vi "Feed Snake.vi"(8 "error in (no error)":errorcluster, 10 "Size":u16, 11 "Snake in":refnum<class "Snake.lvclass">) -> (0 "error out":errorcluster, 3 "Snake out":refnum<class "Snake.lvclass">)   [LabVIEW 2021, in "Snake.lvclass"]
uses:
  Snake.lvclass
  C:/Users/poche/Programs/LabVIEW/imposible snake/GameEl_class/GameEl.lvclass
  GameEl_class/GameEl.lvclass/GameEl.ctl
  GameEl_class/GameEl.lvclass
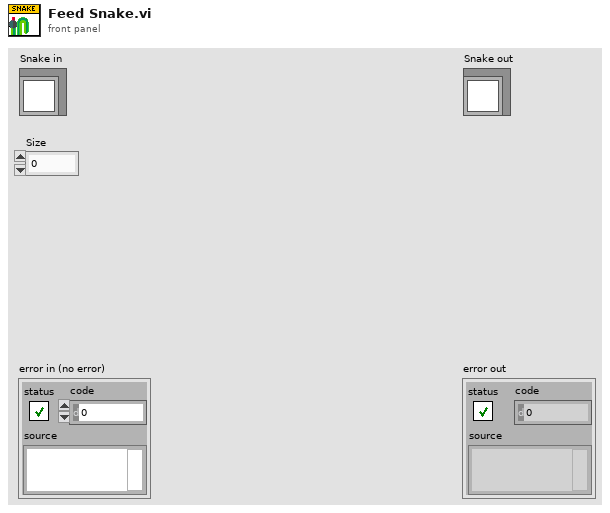
[diagram p1: front panel]
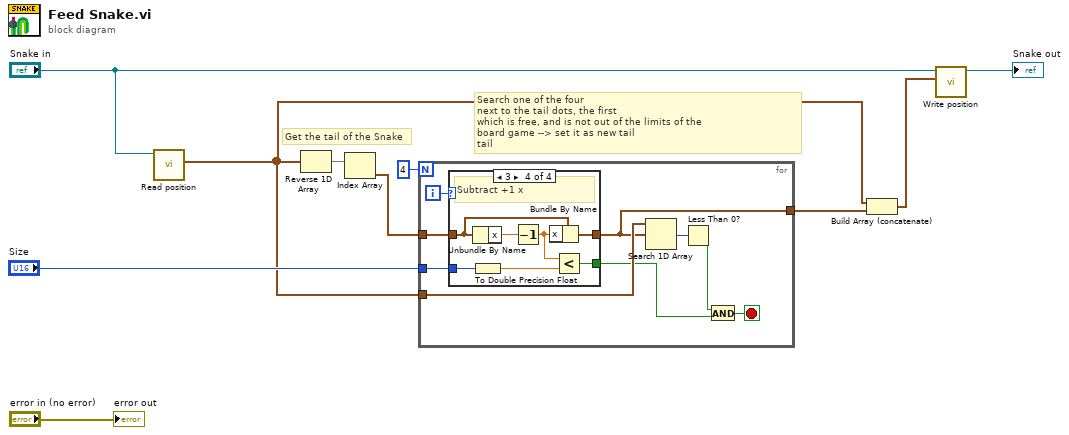
[diagram p0: block diagram]
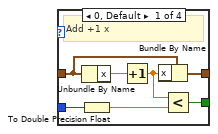
[diagram p2: hidden frame]
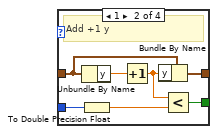
[diagram p3: hidden frame]
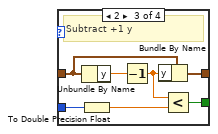
[diagram p4: hidden frame]
diagram:
  # "Search one of the four \nnext to the tail dots, the first \nwhich is free, and is not out of the limits of the \nboard game --> set it as new tail\ntail"
  # "Get the tail of the Snake"
  n1 = call "Read position.vi"("GameEl in"="Snake in") -> ("position"=w4:cluster{"x":dbl, "y":dbl}[])  [unwired: 8 in, 2 out]
  n2 = Reverse 1D Array(array=w4) -> (reversed array=w8:cluster{"x":dbl, "y":dbl}[])
  n3 = Index Array(array=w8) -> (element=w7:cluster{"x":dbl, "y":dbl})  [unwired: 1 in]
  n4 = for {
    N: 4 -> [_]
    tunnel: w7 -> [w19]
    tunnel: w4 -> [w16]
    tunnel: "Size" -> [w17]
    tunnel: [w11] -> w6
    i -> [w18]
    stop <- w12 stop-if-true
    n5 = case shown="3" w18 {
      tunnel: w19 -> [w25 w32 w39 w46]
      tunnel: [w24 w31 w38 w45] -> w11
      tunnel: w17 -> [w22 w29 w36 w43]
      tunnel: [w20 w27 w34 w41] -> w14
      frame 0, Default {
        # "Add +1 x"
        n6 = Unbundle By Name(w25) -> ("x"=w26:dbl)
        n7 = To Double Precision Float(number=w22) -> (double precision float=w21:dbl)
        n8 = Increment(x=w26) -> (x+1=w23:dbl)
        n9 = Bundle By Name(cluster=w25, "x"=w23) -> (w24:cluster{"x":dbl, "y":dbl})
        n10 = Less?(x=w23, y=w21) -> (x < y?=w20:bool)
      }
      frame 1 {
        # "Add +1 y"
        n11 = Unbundle By Name(w32) -> ("y"=w33:dbl)
        n12 = To Double Precision Float(number=w29) -> (double precision float=w28:dbl)
        n13 = Increment(x=w33) -> (x+1=w30:dbl)
        n14 = Bundle By Name(cluster=w32, "y"=w30) -> (w31:cluster{"x":dbl, "y":dbl})
        n15 = Less?(x=w30, y=w28) -> (x < y?=w27:bool)
      }
      frame 2 {
        # "Subtract +1 y"
        n16 = Unbundle By Name(w39) -> ("y"=w40:dbl)
        n17 = To Double Precision Float(number=w36) -> (double precision float=w35:dbl)
        n18 = Decrement(x=w40) -> (x-1=w37:dbl)
        n19 = Bundle By Name(cluster=w39, "y"=w37) -> (w38:cluster{"x":dbl, "y":dbl})
        n20 = Less?(x=w37, y=w35) -> (x < y?=w34:bool)
      }
      frame 3 {
        # "Subtract +1 x"
        n21 = Unbundle By Name(w46) -> ("x"=w47:dbl)
        n22 = To Double Precision Float(number=w43) -> (double precision float=w42:dbl)
        n23 = Decrement(x=w47) -> (x-1=w44:dbl)
        n24 = Bundle By Name(cluster=w46, "x"=w44) -> (w45:cluster{"x":dbl, "y":dbl})
        n25 = Less?(x=w44, y=w42) -> (x < y?=w41:bool)
      }
    }
    n26 = Search 1D Array(1D array=w16, element=w11) -> (index of element=w15:i32)  [unwired: 1 in]
    n27 = Less Than 0?(x=w15) -> (x < 0?=w13:bool)
    n28 = And(x=w13, y=w14) -> (x .and. y?=w12:bool)
  }
  n29 = Build Array (concatenate)(w4, w6) -> (w2:cluster{"x":dbl, "y":dbl}[])
  n30 = call "Write position.vi"("position"=w2, "GameEl in"="Snake in") -> ("GameEl out"=→"Snake out":refnum<class "Snake.lvclass">)  [unwired: 8 in, 1 out]
  "error out" <- "error in (no error)"
